vi "Begin.vi"(8 "error in (no error)":errorcluster, 11 "DriverStation in":refnum<class "DriverStation.lvclass">) -> (0 "error out":errorcluster, 3 "DriverStation out":refnum<class "DriverStation.lvclass">)   [LabVIEW 2013, in "DriverStation.lvclass"]
uses:
  DriverStation.lvclass
  DriverXBoxController/DriverXBoxController.lvclass
  OperatorXBoxController/OperatorXBoxController.lvclass
  System/System.lvclass
  DriverStation.lvclass/DriverStation.ctl
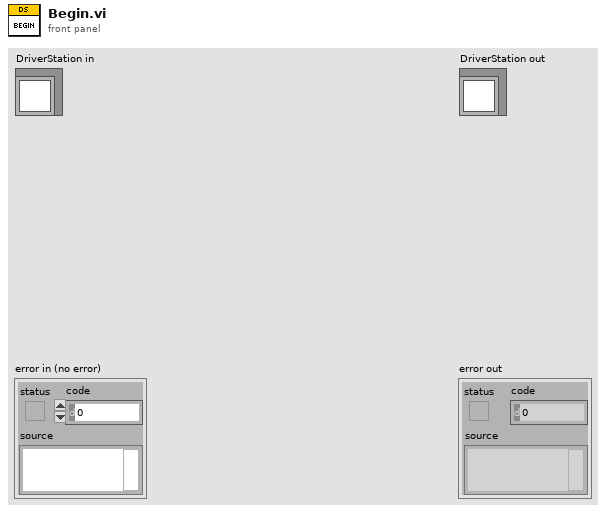
[diagram p1: front panel]
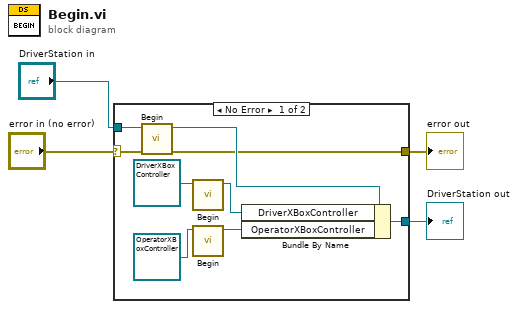
[diagram p0: block diagram]
diagram:
  n1 = case shown="No Error" "error in (no error)" {
    selector: "error in (no error)" -> [w10 w14]
    tunnel: [w9 w14] -> w3
    tunnel: "DriverStation in" -> [w8 w15]
    tunnel: [w7 w15] -> w1
    frame No Error {
      n2 = call-parent "Begin.vi"("error in (no error)"=w10, "System in"=w8) -> ("error out"=w9:errorcluster, "System out"=w11:refnum<class "DriverStation.lvclass">)  [unwired: 8 in]
      n3 = call-dynamic "Begin.vi"("DriverXBoxController in"=refnum<class "DriverXBoxController.lvclass"> refnum ("DriverXBoxController.lvclass")) -> ("DriverXBoxController out"=w13:refnum<class "DriverXBoxController.lvclass">)  [unwired: 9 in, 1 out]
      n4 = call-dynamic "Begin.vi"("OperatorXBoxController in"=refnum<class "OperatorXBoxController.lvclass"> refnum ("OperatorXBoxController.lvclass")) -> ("OperatorXBoxController out"=w5:refnum<class "OperatorXBoxController.lvclass">)  [unwired: 9 in, 1 out]
      n5 = Bundle By Name(cluster=w11, "DriverXBoxController"=w13, "OperatorXBoxController"=w5) -> (w7:refnum<class "DriverStation.lvclass">)
    }
    frame Error {
    }
  }
  "error out" <- w3
  "DriverStation out" <- w1
